vi "Launch Root Actor.vi"(4 "Debug Alias":string, 6 "Open Actor Core front panel? (F)":bool, 8 "error in (no error)":errorcluster, 10 "Actor":refnum<class "Actor.lvclass">) -> (0 "error out":errorcluster, 2 "Actor's Enqueuer":refnum<class "Message Enqueuer.lvclass">)   [LabVIEW 2020, in "Actor Framework.lvlib" / "Actor.lvclass"]
doc: "<p>(<strong>Filename</strong>: <span class=\"dnl\">Actor Framework.lvlib:Actor.lvclass:Launch Root Actor.vi</span>)</p>\n\n<p>Launches an asynchronously running VI that performs tasks and handles messages for the <strong>Actor</strong>. This VI returns a reference to an enqueuer that you can use to send messages to the newly launched actor.</p>\n\n<p>The Launch Root Actor VI launches the <strong>Actor</strong> without a caller. Use this VI to launch the root actor of the actor tree. Use the <a href=\"nihelplauncher://docs/csh?context=lvcore_lvcomm_af_launch_nested_actor\">Launch Nested Actor VI</a> to launch all other actors.</p>"
uses:
  Actor.lvclass
  Message Enqueuer/Message Enqueuer.lvclass
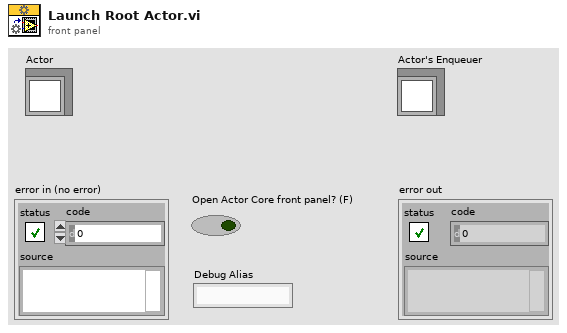
[diagram p1: front panel]
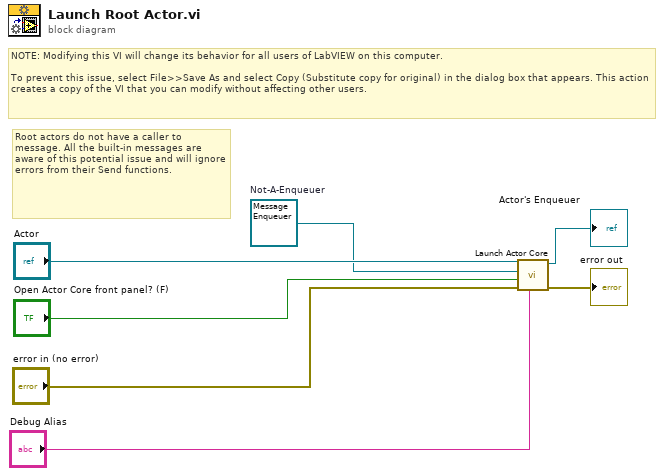
[diagram p0: block diagram]
diagram:
  w2 = refnum<class "Message Enqueuer.lvclass"> refnum  # Not-A-Enqueuer
  # "Root actors do not have a caller to message. All the built-in messages are aware of this potential issue and will ignore errors from their Send functions."
  # "NOTE: Modifying this VI will change its behavior for all users of LabVIEW on this computer.\n\nTo prevent this issue, select File>>Save As and select Copy (Substitute copy for original) in the dialog box that appears. This action creates a copy of the VI that you can modify without affecting other users."
  n1 = call "Launch Actor Core.vi"("Debug Alias"="Debug Alias", "error in (no error)"="error in (no error)", "Open Actor Core front panel?"="Open Actor Core front panel? (F)", "Caller's Enqueuer"=w2, "Actor in"="Actor") -> ("error out"=→"error out":errorcluster, "Message Enqueuer out"=→"Actor's Enqueuer":refnum<class "Message Enqueuer.lvclass">)  [unwired: 5 in]
